vi "ClearableString.vi"(0 "Data In":T4, 2 "Display State In":T2, 3 "Container State":T3) -> (6 "Data Out":T4, 7 "Display State Out":T2, 8 "Action":T1)   [LabVIEW 2011, in "ClearableString.xctl"]
uses:
  ClearableString.xctl
  Data.ctl
  <vilib>/_xctls/Container State.ctl
  State.ctl
  <vilib>/_xctls/Action.ctl
  <vilib>/_xctls/XControlSupport.lvlib
panel:
  in  "Clear":bool
  in  "String":string
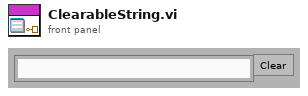
[diagram p1: front panel]
types:
  T1 = typedef "XControlSupport.lvlib/Action.ctl" = cluster{"Data Changed?":bool, "State Changed?":bool, "Action Name":string}
  T2 = typedef "ClearableString.xctl/State.ctl" = cluster{"Numeric":dbl}
  T3 = typedef "XControlSupport.lvlib/Container State.ctl" = cluster{"Indicator?":bool, "Run Mode?":bool, " Refnum":refnum<vi>}
  T4 = typedef "ClearableString.xctl/Data.ctl" = string
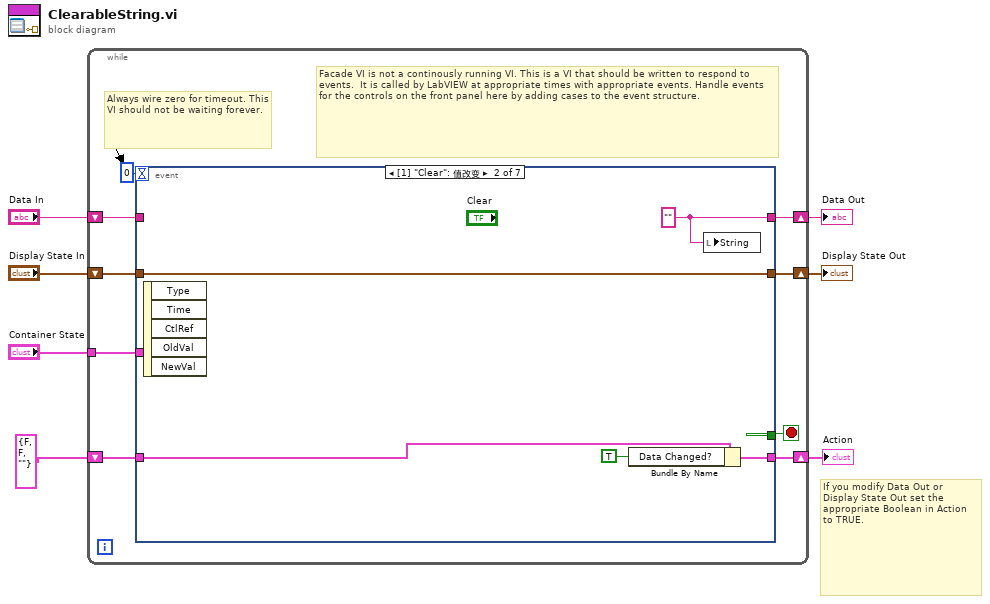
[diagram p0: block diagram]
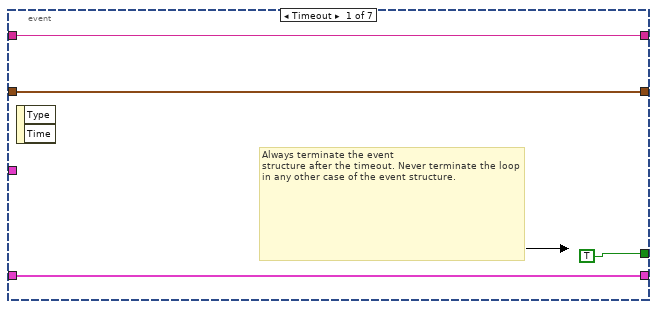
[diagram p2: hidden frame]
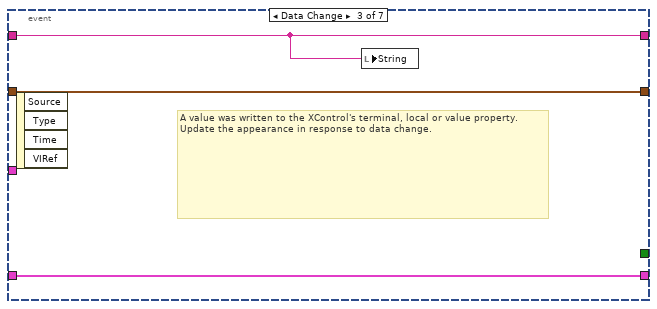
[diagram p3: hidden frame]
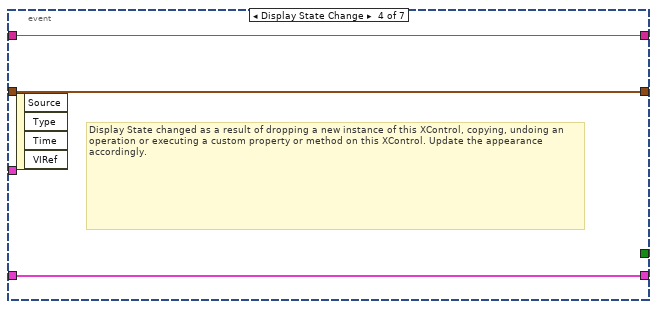
[diagram p4: hidden frame]
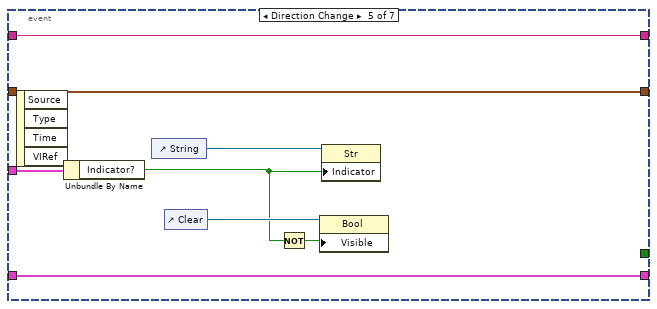
[diagram p5: hidden frame]
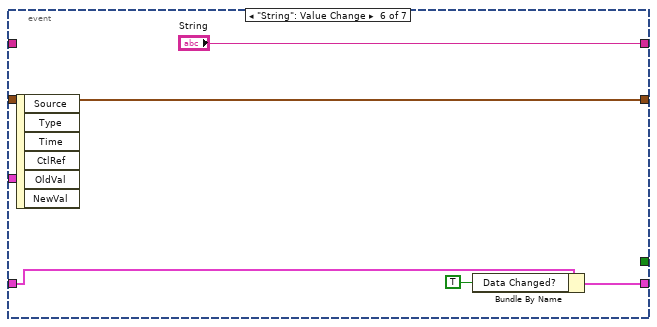
[diagram p6: hidden frame]
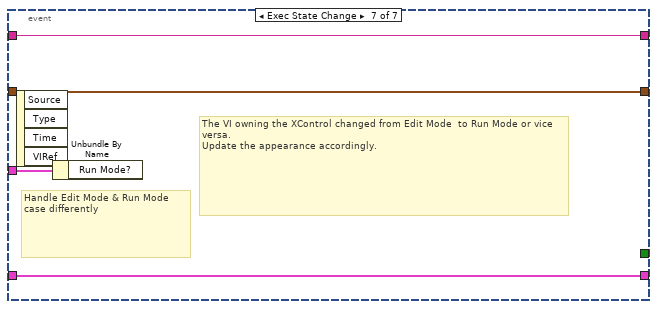
[diagram p7: hidden frame]
diagram:
  # "If you modify Data Out or\nDisplay State Out set the\nappropriate Boolean in Action\nto TRUE."
  n1 = while {
    shift-right: [w15] -> w4
    shift-left: "Display State In" -> [w16]
    tunnel: "Container State" -> [w12]
    shift-right: [w10] -> w7
    shift-left: "Data In" -> [w11]
    shift-right: [w8] -> w2
    shift-left: T1 {"Data Changed?"=FALSE, "State Changed?"=FALSE, "Action Name"=""} ("Action") -> [w9]
    stop <- w14 stop-if-true
    # "Facade VI is not a continously running VI. This is a VI that should be written to respond to events.  It is called by LabVIEW at appropriate times with appropriate events. Handle events for the controls on the front panel here by adding cases to the event structure."
    # "Always wire zero for timeout. This\nVI should not be waiting forever."
    n2 = event shown="[1] \"Clear\": 值改变" {
      selector: _ -> [_ _ _ _ _ _ _]
      dyn-events: _ -> [_ _ _ _ _ _ _]
      timeout: 0 -> [_ _ _ _ _ _ _]
      tunnel: w16 -> [w18 w25 w28 w31 w38 w43 w47]
      tunnel: [w18 w25 w28 w31 w38 w43 w47] -> w15
      tunnel: [TRUE _ _ _ _ _ _] -> w14
      tunnel: w12 -> [_ _ _ _ w39 _ w48]
      tunnel: w11 -> [w17 _ w26 w30 w37 _ w46]
      tunnel: [w17 w21 w26 w30 w37 "String" w46] -> w10
      tunnel: [w19 w24 w27 w29 w36 w42 w45] -> w8
      tunnel: w9 -> [w19 w23 w27 w29 w36 w41 w45]
      event Timeout {
        # "Always terminate the event\nstructure after the timeout. Never terminate the loop in any other case of the event structure."
        n3 = event-data() -> ()  [unwired: 1 in, 2 out]
      }
      event "Clear": Value Change {
        w21 = T4 "" ("t")
        n4 = event-data() -> ()  [unwired: 1 in, 5 out]
        n5 = Bundle By Name(cluster=w23, "Data Changed?"=TRUE) -> (w24:T1)
        n6 = local write "String"(w21) -> ()
      }
      event Data Change {
        # "A value was written to the XControl's terminal, local or value property.\nUpdate the appearance in response to data change."
        n7 = event-data() -> ()  [unwired: 1 in, 4 out]
        n8 = local write "String"(w26) -> ()
      }
      event Display State Change {
        # "Display State changed as a result of dropping a new instance of this XControl, copying, undoing an operation or executing a custom property or method on this XControl. Update the appearance accordingly."
        n9 = event-data() -> ()  [unwired: 1 in, 4 out]
      }
      event Direction Change {
        n10 = event-data() -> ()  [unwired: 1 in, 4 out]
        n11 = Unbundle By Name(w39) -> ("Indicator?"=w33:bool)
        n12 = control-ref of="String"() -> (w35:refnum<vi>)
        n13 = control-ref of="Clear"() -> (w34:refnum<vi>)
        n14 = Not(x=w33) -> (.not. x?=w32:bool)
        n15 = property class="Bool"(reference=w34, "Visible"=w32) -> ()  [unwired: 1 in, 2 out]
        n16 = property class="Str"(reference=w35, "Indicator"=w33) -> ()  [unwired: 1 in, 2 out]
      }
      event "String": Value Change {
        n17 = event-data() -> ()  [unwired: 1 in, 6 out]
        n18 = Bundle By Name(cluster=w41, "Data Changed?"=TRUE) -> (w42:T1)
      }
      event Exec State Change {
        # "The VI owning the XControl changed from Edit Mode  to Run Mode or vice versa.\nUpdate the appearance accordingly."
        # "Handle Edit Mode & Run Mode\ncase differently"
        n19 = event-data() -> ()  [unwired: 1 in, 4 out]
        n20 = Unbundle By Name(w48) -> ()  [unwired: 1 out]
      }
    }
  }
  "Display State Out" <- w4
  "Data Out" <- w7
  "Action" <- w2
